vi "Acquisition Message Loop.vi"(8 "error in (no error)":cluster{"状态":bool, "代码":i32, "源":string} caption="错误输入（无错误）", 9 "数据队列":refnum<queue>, 10 "数据通知器":refnum<notifier>, 11 "消息队列":T1) -> (0 "error out":cluster{"状态":bool, "代码":i32, "源":string} caption="错误输出")   [LabVIEW 2014, in "Acquisition.lvlib"]
doc: "该消息循环负责处理硬件数据采集的相关消息。"
uses:
  Acquisition.lvlib
  support/Message Queue/All Message Queues.ctl
  support/Message Queue/Message Cluster.ctl
  Hardware Configuration.ctl
  Signal Type.ctl
  Acquisition State.ctl
  support/Message Queue/Enqueue Message (Single).vi
  <vilib>/Utility/error.llb/Error Cluster From Error Code.vi
  <vilib>/ErrorRing/Error Ring.xnode
  support/Message Queue/Message Queue.lvlib
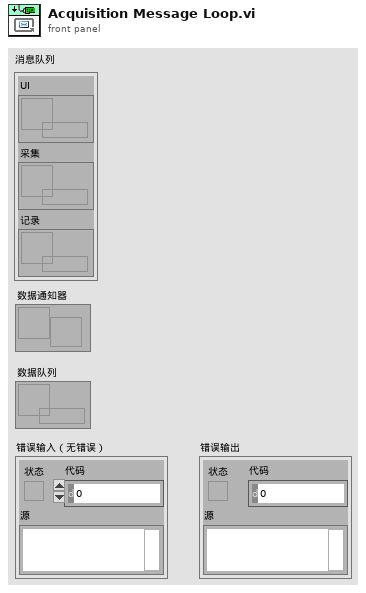
[diagram p1: front panel]
types:
  T1 = typedef "Message Queue.lvlib/All Message Queues.ctl" = cluster{"UI":refnum<queue>, "采集":refnum<queue>, "记录":refnum<queue>}
  T2 = typedef "Acquisition.lvlib/Hardware Configuration.ctl" = cluster{"硬件引用句柄<替换此项>":string, "信号类型<替换该项>":T3}
  T3 = typedef "Acquisition.lvlib/Signal Type.ctl" = enum16{"Sine Wave", "Square with Noise"}
  T4 = typedef "Acquisition.lvlib/Acquisition State.ctl" = enum16{"Idle", "Acquiring"}
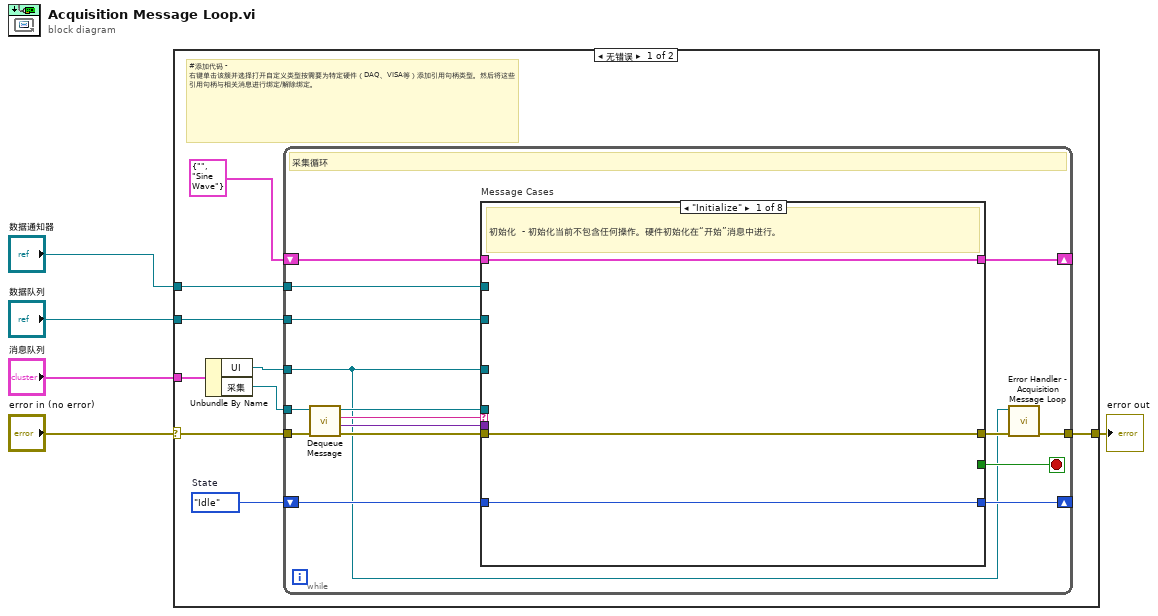
[diagram p0: block diagram]
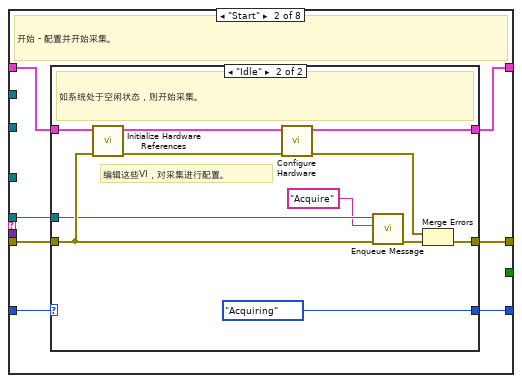
[diagram p2: hidden frame]
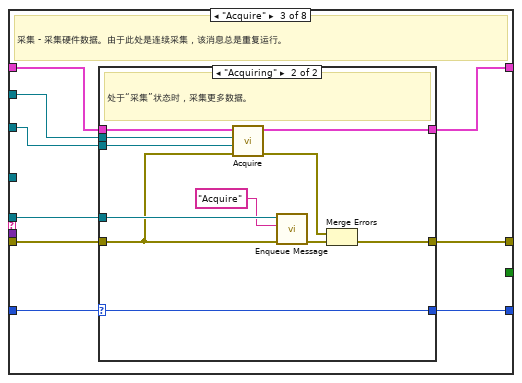
[diagram p4: hidden frame]
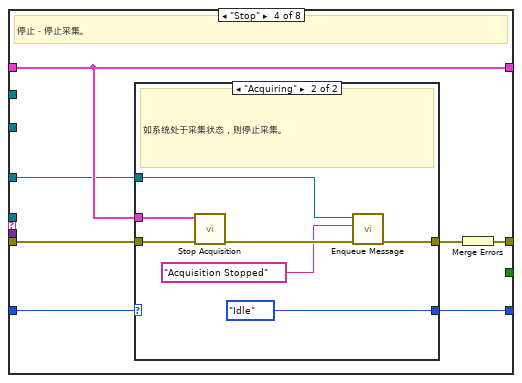
[diagram p6: hidden frame]
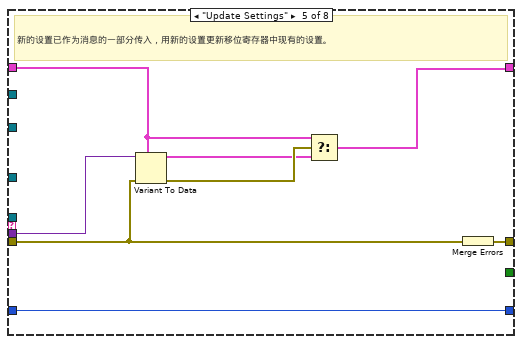
[diagram p8: hidden frame]
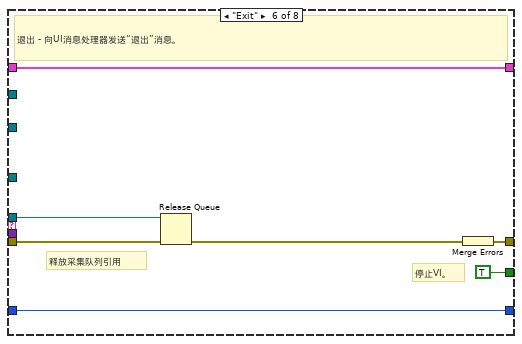
[diagram p9: hidden frame]
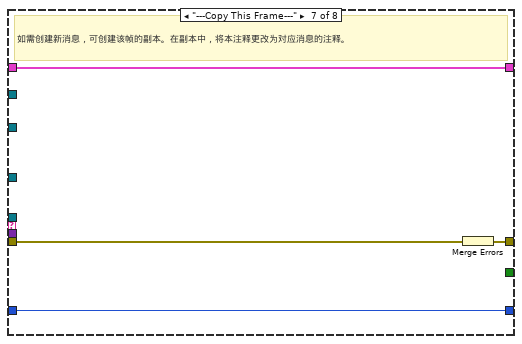
[diagram p10: hidden frame]
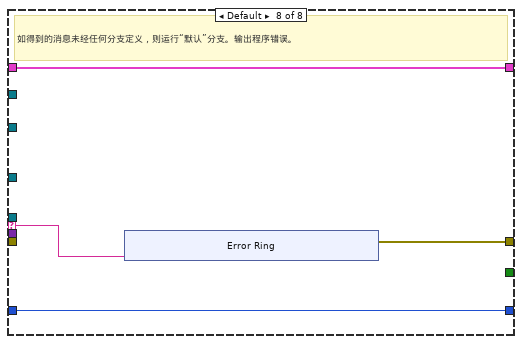
[diagram p11: hidden frame]
diagram:
  n1 = case shown="无错误" "error in (no error)" {
    selector: "error in (no error)" -> [w10 w124]
    tunnel: "消息队列" -> [w14 _]
    tunnel: [w12 w124] -> w4
    tunnel: "数据通知器" -> [w8 _]
    tunnel: "数据队列" -> [w7 _]
    frame No Error {
      w6 = Acquisition_State."Idle"  # State
      # "#添加代码 - 右键单击该簇并选择打开自定义类型按需要为特定硬件（DAQ、VISA等）添加引用句柄类型。然后将这些引用句柄与相关消息进行绑定/解除绑定。"
      n2 = Unbundle By Name(w14) -> ("UI"=w9:refnum<queue>, "采集"=w13:refnum<queue>)
      n3 = while {
        tunnel: w13 -> [w23]
        shift-right: [w29] -> _
        shift-left: T2 {"硬件引用句柄<替换此项>"="", "信号类型<替换该项>"=enum."Sine Wave"} ("Data Cluster") -> [w30]
        tunnel: w9 -> [w15]
        tunnel: w8 -> [w22]
        tunnel: w7 -> [w21]
        shift-right: [w19] -> _
        shift-left: w6 -> [w20]
        tunnel: w10 -> [w27]
        tunnel: [w18] -> w12
        stop <- w28 stop-if-true
        # "采集循环"
        n4 = call "Dequeue Message.vi"("error in (no error)"=w27, "消息队列"=w23) -> ("error out"=w26:cluster{"状态":bool, "代码":i32, "源":string}, "消息数据"=w24:variant, "消息"=w25:string, "消息队列副本"=w16:refnum<queue>)  [unwired: 6 in]
        n5 = case "Message Cases" shown="\"Initialize\"" w25 {
          selector: w25 -> [_ _ _ _ _ _ _ w113]
          tunnel: w16 -> [_ w37 w62 _ _ w103 _ _]
          tunnel: w26 -> [w33 w38 w61 w83 w95 w105 w112 _]
          tunnel: [w33 w40 w63 w84 w101 w107 w110 w114] -> w17
          tunnel: w30 -> [w32 w39 w59 w81 w97 w106 w111 w116]
          tunnel: [w32 w36 w60 w81 w96 w106 w111 w116] -> w29
          tunnel: [_ _ _ _ _ TRUE _ _] -> w28
          tunnel: w24 -> [_ _ _ _ w100 _ _ _]
          tunnel: w15 -> [_ _ _ w78 _ _ _ _]
          tunnel: w22 -> [_ _ w58 _ _ _ _ _]
          tunnel: w21 -> [_ _ w57 _ _ _ _ _]
          tunnel: w20 -> [w31 w34 w55 w80 w94 w102 w109 w115]
          tunnel: [w31 w35 w56 w79 w94 w102 w109 w115] -> w19
          frame "Initialize" {
            # "初始化  - 初始化当前不包含任何操作。硬件初始化在“开始”消息中进行。"
          }
          frame "Start" {
            # "开始 - 配置并开始采集。"
            n6 = case shown="\"Idle\"" w34 {
              selector: w34 -> [w41 _]
              tunnel: [w42 w54] -> w40
              tunnel: w39 -> [w43 w53]
              tunnel: w38 -> [w42 w52]
              tunnel: w37 -> [_ w50]
              tunnel: [w43 w46] -> w36
              tunnel: [w41 Acquisition_State."Acquiring" ("Acquisition State")] -> w35
              frame "Acquiring" {
                # "系统已开始采集。忽略“开始”消息。"
              }
              frame "Idle" {
                # "编辑这些VI，对采集进行配置。"
                # "如系统处于空闲状态，则开始采集。"
                n7 = call "Initialize Hardware References.vi"("error in (no error)"=w52, "硬件资源输入"=w53) -> ("error out"=w49:cluster{"状态":bool, "代码":i32, "源":string}, "硬件资源输出"=w47:T2)  [unwired: 8 in]
                n8 = call "Configure Hardware.vi"("error in (no error)"=w49, "硬件资源输入"=w47) -> ("error out"=w48:cluster{"状态":bool, "代码":i32, "源":string}, "硬件资源输出"=w46:T2)  [unwired: 8 in]
                n9 = call-poly "Enqueue Message.vi"("error in (no error)"=w52, "消息"="Acquire" ("Message"), "消息队列"=w50) -> ("error out"=w51:cluster{"状态":bool, "代码":i32, "源":string})  [unwired: 7 in, 1 out]
                n10 = Merge Errors(w48, w51) -> (w54:errorcluster)
              }
            }
          }
          frame "Acquire" {
            # "采集 - 采集硬件数据。由于此处是连续采集，该消息总是重复运行。"
            n11 = case shown="\"Acquiring\"" w55 {
              selector: w55 -> [w64 w68]
              tunnel: [w65 w77] -> w63
              tunnel: w62 -> [_ w75]
              tunnel: w61 -> [w65 w67]
              tunnel: [w66 w73] -> w60
              tunnel: w59 -> [w66 w72]
              tunnel: w58 -> [_ w70]
              tunnel: w57 -> [_ w69]
              tunnel: [w64 w68] -> w56
              frame "Idle" {
                # "如采集处于空闲状态，则忽略“采集”消息。"
              }
              frame "Acquiring" {
                # "处于“采集”状态时，采集更多数据。"
                n12 = call "Acquire.vi"("error in (no error)"=w67, "数据队列"=w69, "数据通知器"=w70, "硬件资源输入"=w72) -> ("error out"=w74:cluster{"状态":bool, "代码":i32, "源":string}, "硬件资源输出"=w73:T2)  [unwired: 6 in]
                n13 = call-poly "Enqueue Message.vi"("error in (no error)"=w67, "消息"="Acquire" ("Message"), "消息队列"=w75) -> ("error out"=w76:cluster{"状态":bool, "代码":i32, "源":string})  [unwired: 7 in, 1 out]
                n14 = Merge Errors(w74, w76) -> (w77:errorcluster)
              }
            }
          }
          frame "Stop" {
            # "停止－停止采集。"
            n15 = case shown="\"Acquiring\"" w80 {
              selector: w80 -> [w85 _]
              tunnel: w83 -> [w86 w93]
              tunnel: [w86 w89] -> w82
              tunnel: w81 -> [_ w91]
              tunnel: [w85 Acquisition_State."Idle" ("State")] -> w79
              tunnel: w78 -> [_ w88]
              frame "Idle" {
                # "系统已处于空闲状态。忽略“停止”消息。"
              }
              frame "Acquiring" {
                # "如系统处于采集状态，则停止采集。"
                n16 = call "Stop Acquisition.vi"("error in (no error)"=w93, "硬件资源输入"=w91) -> ("error out"=w92:cluster{"状态":bool, "代码":i32, "源":string})  [unwired: 9 in]
                n17 = call-poly "Enqueue Message.vi"("error in (no error)"=w92, "消息"="Acquisition Stopped", "消息队列"=w88) -> ("error out"=w89:cluster{"状态":bool, "代码":i32, "源":string})  [unwired: 7 in, 1 out]
              }
            }
            n18 = Merge Errors(w82) -> (w84:errorcluster)
          }
          frame "Update Settings" {
            # "新的设置已作为消息的一部分传入，用新的设置更新移位寄存器中现有的设置。"
            n19 = Variant To Data(error in=w95, type=w97, Variant=w100) -> (data=w98:T2, error out=w99:errorcluster)
            n20 = Select(t=w97, s=w99, f=w98) -> (s? t:f=w96:T2)
            n21 = Merge Errors(w95) -> (w101:errorcluster)
          }
          frame "Exit" {
            # "释放采集队列引用"
            # "停止VI。"
            # "退出 - 向UI消息处理器发送“退出”消息。"
            n22 = Release Queue(queue=w103, error in (no error)=w105) -> (error out=w104:errorcluster)  [unwired: 1 in, 2 out]
            n23 = Merge Errors(w104) -> (w107:errorcluster)
          }
          frame "---Copy This Frame---" {
            # "如需创建新消息，可创建该帧的副本。在副本中，将本注释更改为对应消息的注释。"
            n24 = Merge Errors(w112) -> (w110:errorcluster)
          }
          frame Default {
            # "如得到的消息未经任何分支定义，则运行“默认”分支。输出程序错误。"
            n25 = xnode "Error Ring"("参数 0"=w113) -> ("错误输出"=w114:errorcluster)
          }
        }
        n26 = call "Error Handler - Acquisition Message Loop.vi"("error in (no error)"=w17, "消息队列"=w15) -> ("错误输入副本"=w18:cluster{"状态":bool, "代码":i32, "源":string})  [unwired: 8 in, 1 out]
      }
    }
    frame Error {
    }
  }
  "error out" <- w4
